vi "State_Machine.vi"(8 "error in (no error)":errorcluster caption="entrée d'erreur (pas d'erreur)", 11 "Send_Frame en entrée":refnum<class "Nodon_Read_Event_UART.lvclass">) -> (0 "error out":errorcluster caption="sortie d'erreur", 2 "Json_String":string, 3 "Send_Frame en sortie":refnum<class "Nodon_Read_Event_UART.lvclass">)   [LabVIEW 2020, in "Library Test.lvlib" / "Nodon_Read_Event_UART.lvclass"]
uses:
  Nodon_Read_Event_UART.lvclass
  JSON API/Variant JSON/Variant to JSON.vi
  JSON API/JSON Value/Get Item by name array.vi
  JSON API/JSON Value/JSON Value.lvclass
  Nodon_Read_Event_UART.lvclass/Nodon_Read_Event_UART.ctl
  JSON API/Get Polymorphic/JSON GetSet.lvlib
  JSON API/Variant JSON/Variant JSON.lvlib
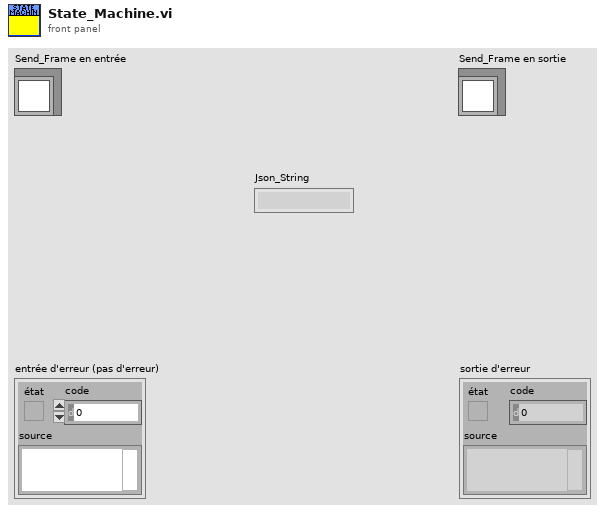
[diagram p1: front panel]
types:
  T1 = cluster{"Commande Type":string, "Command ID":string, "Data":string, "Error":string}
  T2 = enum16{"Empty port", "Send Frame", "Wait Return Ack", "Wait Return Report", "Check End", "End"}
  T3 = enum16{"Empty port", "Send Frame", "Wait Return Ack", "Wait Return Report", "Check End"}
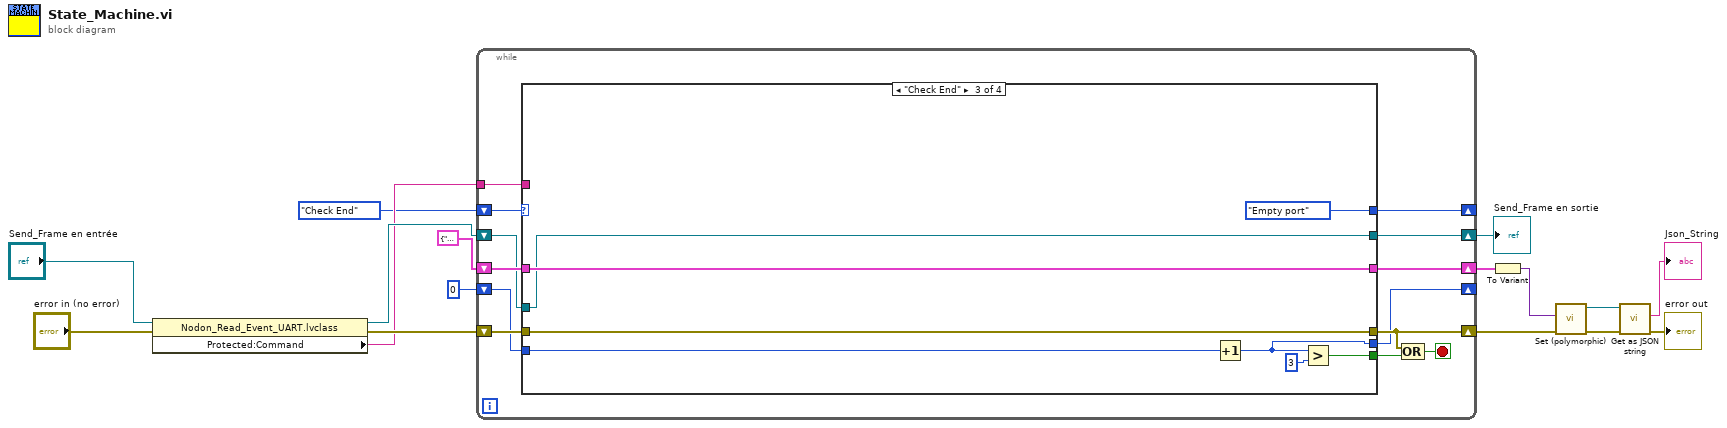
[diagram p0: block diagram]
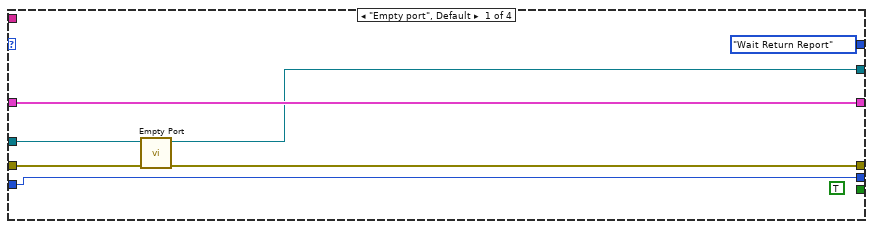
[diagram p2: hidden frame]
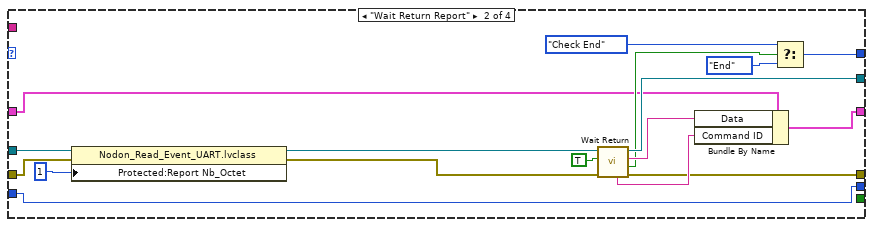
[diagram p3: hidden frame]
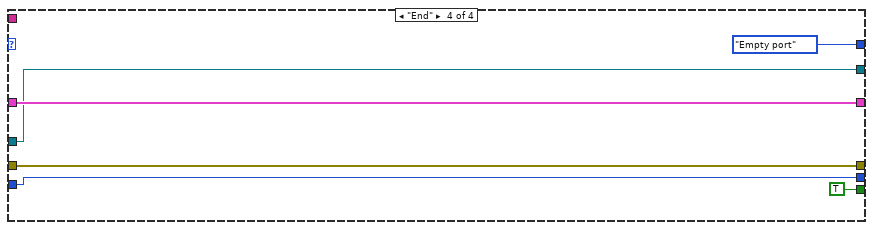
[diagram p4: hidden frame]
diagram:
  n1 = property class="Nodon_Read_Event_UART.lvclass"(reference="Send_Frame en entrée", error in="error in (no error)") -> (reference out=w14:refnum<class "Nodon_Read_Event_UART.lvclass">, error out=w13:errorcluster, "Protected:Command"=w11:string)
  n2 = while {
    tunnel: w11 -> [w28]
    shift-right: [w29] -> w15
    shift-left: w14 -> [w22]
    shift-right: [w21] -> w3
    shift-left: w13 -> [w27]
    shift-right: [w26] -> _
    shift-left: T2."Check End" -> [w25]
    shift-right: [w23] -> w2
    shift-left: T1 {"Commande Type"="", "Command ID"="", "Data"="", "Error"=""} -> [w24]
    shift-right: [w17] -> _
    shift-left: 0 -> [w19]
    stop <- w20 stop-if-true
    n3 = case shown="\"Check End\"" w25 {
      tunnel: [w35 w47 w61 w67] -> w21
      tunnel: [w32 w53 w58 w64] -> w29
      tunnel: w28 -> [_ _ _ _]
      tunnel: w27 -> [w36 w46 w61 w67]
      tunnel: [T2."Wait Return Report" w52 T3."Empty port" T3."Empty port"] -> w26
      tunnel: w24 -> [w34 w37 w59 w65]
      tunnel: [w34 w48 w59 w65] -> w23
      tunnel: w22 -> [w33 w45 w58 w64]
      tunnel: w19 -> [w30 w39 w55 w62]
      tunnel: [_ _ w56 TRUE] -> w18
      tunnel: [w30 w39 w54 w62] -> w17
      frame "Empty port", Default {
        (unwired) TRUE ("Frame NOk")
        n4 = call-dynamic "Empty Port.vi"("entrée d'erreur (pas d'erreur)"=w36, "Send_Frame en entrée"=w33) -> ("sortie d'erreur"=w35:errorcluster, "Send_Frame en sortie"=w32:refnum<class "Nodon_Read_Event_UART.lvclass">)  [unwired: 8 in]
      }
      frame "Wait Return Report" {
        n5 = property class="Nodon_Read_Event_UART.lvclass"(reference=w45, error in=w46, "Protected:Report Nb_Octet"=u16 1 ("Report Nb_Octet")) -> (reference out=w44:refnum<class "Nodon_Read_Event_UART.lvclass">, error out=w38:errorcluster)
        n6 = call-dynamic "Wait Return.vi"("entrée d'erreur (pas d'erreur)"=w38, "Report ?"=TRUE ("Report"), "Send_Frame en entrée"=w44) -> ("sortie d'erreur"=w47:errorcluster, "Send again"=w42:bool, "Data"=w49:string, "Send_Frame en sortie"=w53:refnum<class "Nodon_Read_Event_UART.lvclass">, "Command ID"=w50:string)  [unwired: 3 in, 1 out]
        n7 = Bundle By Name(cluster=w37, "Data"=w49, "Command ID"=w50) -> (w48:T1)
        n8 = Select(t=T2."Check End", s=w42, f=T2."End") -> (s? t:f=w52:T2)
      }
      frame "Check End" {
        n9 = Increment(x=w55) -> (x+1=w54:i32)
        n10 = Greater?(x=w54, y=3) -> (0:w56:bool)
      }
      frame "End" {
      }
    }
    n11 = Compound Arithmetic op=OR ("Opérateur arithmétique")(w21, w18) -> (w20:bool)
  }
  "Send_Frame en sortie" <- w15
  n12 = To Variant(anything=w2) -> (Variant=w4:variant)
  n13 = call-poly "Set (polymorphic).vi"("error in (no error)"=w3, "Variant"=w4) -> ("error out"=w6:errorcluster, "JSON Value out"=w5:refnum<class "JSON Value.lvclass">)  [unwired: 8 in]
  n14 = call "Get as JSON string.vi"("error in (no error)"=w6, "JSON Value in"=w5) -> ("error out"=→"error out":errorcluster, "<JSON>"=→"Json_String":string)  [unwired: 8 in]
